vi "Display Module.vi"(8 "error in":errorcluster) -> (0 "error out":errorcluster)   [LabVIEW 2018, in "Display.lvlib"]
doc: "This is the top level of the wash display module (a free running module of the Car WAsh simulator). \n\nIt is closed using a user event. It communicates with the other modules using a queue based API which has comms modules that can be swapped if required."
uses:
  Display.lvlib
  Private Controls/Module Action.ctl
  Private Controls/Module Data Cluster.ctl
  Entry Console/Entry Console/Public Controls/Entry Console.ctl
  Entry Console/Entry Console/Entry Console.lvlib
  public controls/Display Data.ctl
panel:
  out "Time Remaining":dbl format="%07.2f seconds"
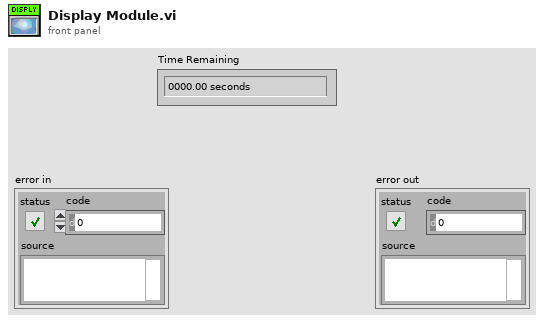
[diagram p1: front panel]
types:
  T1 = typedef "Display.lvlib/Display Data.ctl" = cluster{"Variant":variant}
  T2 = typedef "Display.lvlib/Module Data Cluster.ctl" = cluster{"Variant":variant, "action":T3}
  T3 = typedef "Display.lvlib/Module Action.ctl" = enum16{"error", "exit", "init", "Update Display"}
  T4 = cluster{"Variant":variant, "action":enum16{"error", "exit", "init"}}
  T5 = typedef "Entry Console.lvlib/Wash Step Selection Buttons.ctl" = cluster{"Under Body Wash":bool, "Bug Remover":bool, "Pre-Soak":bool, "High Pressure Wash":bool, "Low Pressure Wax":bool, "Spot Free Rinse":bool, "Tire Shine Foam":bool, "Air Dry":bool}
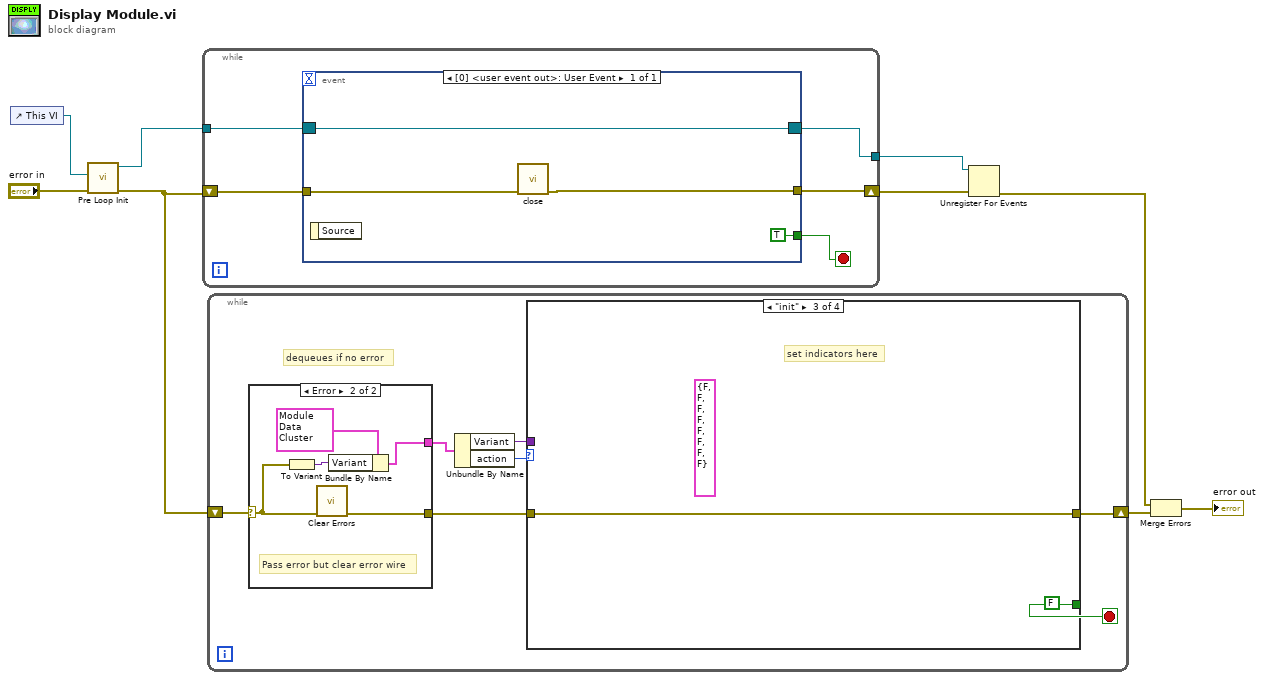
[diagram p0: block diagram]
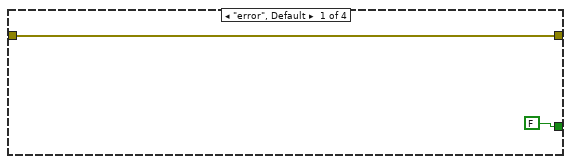
[diagram p2: hidden frame]
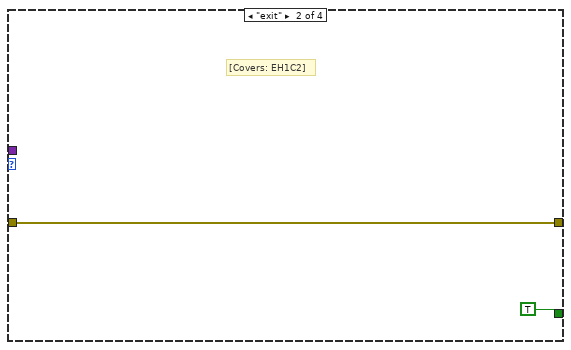
[diagram p3: hidden frame]
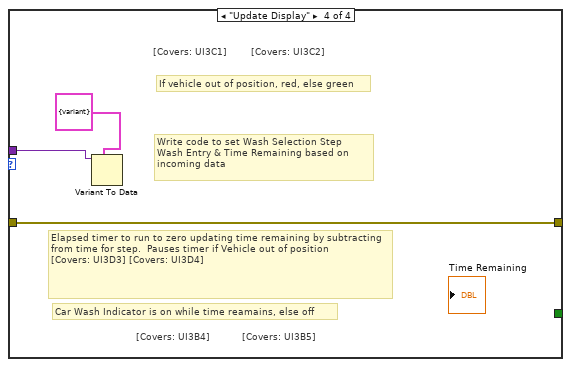
[diagram p4: hidden frame]
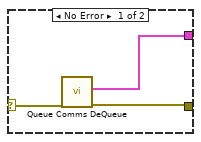
[diagram p5: hidden frame]
diagram:
  n1 = control-ref of="This VI"() -> (w9:refnum<vi>)
  n2 = call "Pre Loop Init.vi"("error in"="error in", "Ref In"=w9) -> ("error out"=w6:errorcluster, "Event Registration Refnum"=w8:refnum<event-registration>)  [unwired: 8 in]
  n3 = while {
    shift-right: [w13] -> w5
    shift-left: w6 -> [w14]
    tunnel: w8 -> [w12]
    tunnel: [w10] -> w4
    stop <- w11 stop-if-true
    n4 = event shown="[0] <user event out>: User Event" {
      selector: w12 -> [w15]
      dyn-events: [w15] -> w10
      timeout: _ -> [_]
      tunnel: w14 -> [w18]
      tunnel: [w17] -> w13
      tunnel: [TRUE] -> w11
      event User Event {
        n5 = event-data() -> ()  [unwired: 1 in, 1 out]
        n6 = call "close.vi"("error in"=w18) -> ("error out"=w17:errorcluster)  [unwired: 10 in]
      }
    }
  }
  n7 = while {
    shift-right: [w21] -> w3
    shift-left: w6 -> [w25]
    stop <- w19 stop-if-true
    # "dequeues if no error"
    n8 = case shown="Error" w25 {
      selector: w25 -> [w37 w42]
      tunnel: [w36 w38] -> w24
      tunnel: [w35 w41] -> w20
      frame No Error {
        n9 = call "Queue Comms DeQueue.vi"("error in"=w37) -> ("error out"=w35:errorcluster, "element"=w36:T4)  [unwired: 9 in]
      }
      frame Error {
        # "Pass error but clear error wire"
        n10 = To Variant(anything=w42) -> (Variant=w39:variant)
        n11 = call <vilib>:"Clear Errors.vi"("error in (no error)"=w42) -> ("error out"=w41:errorcluster)  [unwired: 5 in, 1 out]
        n12 = Bundle By Name(cluster=T2 {"Variant"=variant, "action"=enum."error"} ("element"), "Variant"=w39) -> (w38:T2)
      }
    }
    n13 = Unbundle By Name(w24) -> ("Variant"=w22:variant, "action"=w23:T3)
    n14 = case shown="\"init\"" w23 {
      tunnel: w22 -> [_ _ _ w33]
      tunnel: [w27 w29 w31 w34] -> w21
      tunnel: w20 -> [w27 w29 w31 w34]
      tunnel: [FALSE TRUE FALSE _] -> w19
      frame "error", Default {
      }
      frame "exit" {
        # "[Covers: EH1C2]"
      }
      frame "init" {
        (unwired) T5 {"Under Body Wash"=FALSE, "Bug Remover"=FALSE, "Pre-Soak"=FALSE, "High Pressure Wash"=FALSE, "Low Pressure Wax"=FALSE, "Spot Free Rinse"=FALSE, "Tire Shine Foam"=FALSE, "Air Dry"=FALSE} ("WashStepSelection")
        # "set indicators here"
      }
      frame "Update Display" {
        # "Car Wash Indicator is on while time reamains, else off"
        # "[Covers: UI3C2]"
        # "[Covers: UI3C1]"
        # "If vehicle out of position, red, else green"
        # "[Covers: UI3B5]"
        # "[Covers: UI3B4]"
        # "Elapsed timer to run to zero updating time remaining by subtracting from time for step.  Pauses timer if Vehicle out of position\n[Covers: UI3D3] [Covers: UI3D4]"
        # "Write code to set Wash Selection Step\nWash Entry & Time Remaining based on \nincoming data"
        n15 = Variant To Data(type=T1 {"Variant"=variant}, Variant=w33) -> ()  [unwired: 1 in, 2 out]
      }
    }
  }
  n16 = Unregister For Events(event registration refnum=w4, error in=w5) -> (error out=w1:errorcluster)
  n17 = Merge Errors(w1, w3) -> (→"error out":errorcluster)
